vi "Trap2-TestRT-05-16.vi"() -> ()   [LabVIEW 2010]
uses:
  <vilib>/userDefined/High Color/nirio_resource_hc.ctl
  <vilib>/rvi/interface/nirviOpenFPGA/nirviOpenFPGA.xnode
  C:/Users/HAGAR-IV/Desktop/Zeugs/markus/version feb 2012/FPGA Bitfiles/pertrasgcfpga2_FPGATarget_Trap2-Test-05-16_C889B2AB.lvbitx
  C:/Users/HAGAR-IV/Desktop/HAGAR-V_Steuerung/Users/HAGAR-IV/Desktop/Johnny/pertrasgc fpga/Trap2-Test-05-16.vi
  <vilib>/rvi/ClientSDK/nirviWhatTheDeviceIsDoing.ctl
  <vilib>/rvi/interface/nirviReadWriteControl/nirviReadWriteControl.xnode
  <vilib>/rvi/interface/common/niFpgaNodeNameForErrorReporting.ctl
  <vilib>/rvi/errors/niLvFpgaWhatHappensToTopLevelVI.ctl
  <vilib>/rvi/interface/nirviMethod/nirviMethod.xnode
  <vilib>/rvi/interface/nirviCloseFPGA/nirviCloseFPGA.xnode
  <vilib>/FPGAPlugInAG/cRIO-9114/niLvFpga_Open_cRIO-9114.vi
  <vilib>/rvi/interface/common/dynamic/niFpgaDynamicAddResources.vi
  <vilib>/Utility/error.llb/Error Cluster From Error Code.vi
  <vilib>/rvi/errors/niLvFpgaAdjustHostInterfaceError.vi
  <vilib>/FPGAPlugInAG/Dynamic/niLvFpga_Close_Dynamic.vi
  NiFpgaLv.dll
panel:
  out "XY Graph":cluster{dbl[], dbl[]}(graph)
  out "UTempMax":fxp<+/-,16,4> format="%.14g"
  out "UTemp":fxp<+/-,16,4> format="%.14g"
  out "UTempSP":fxp<+/-,16,4> format="%.14g"
  in  "Traps/MachKoeff":dbl[](array[numeric])
  out "UTemp[V]Trap2":dbl format="%.14g"
  in  "stop":bool
  in  "Per[us]Trap2":u32
  in  "warten[us]Trap2":u32
  in  "UTempSPTrap2":dbl format="%.14g"
  in  "UTempMaxTrap2":dbl format="%.14g"
  in  "PIDTrap2":T1 {"proportional gain (Kc)" format="%.11g"; "integral gain (Kc*Ts/Ti)" format="%.11g"; "derivative gain (Kc*Td/Ts)" format="%.11g"}
  in  "Heizen?Trap2":bool
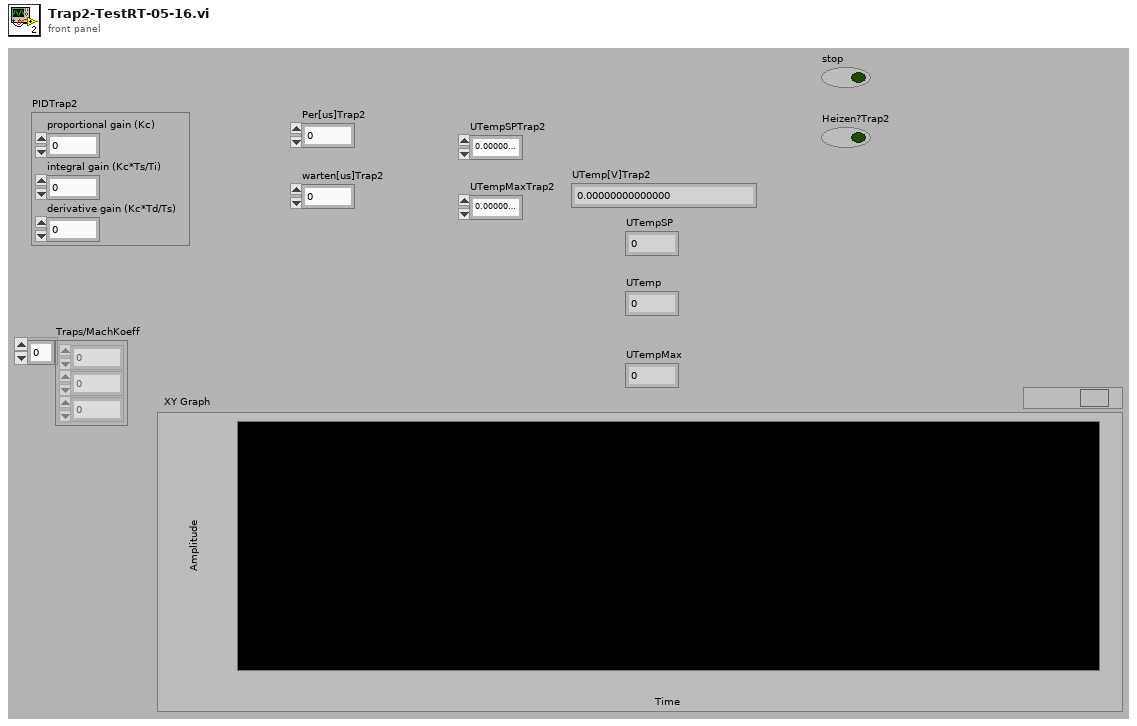
[diagram p1: front panel]
types:
  T1 = cluster{"proportional gain (Kc)":fxp<+/-,16,8>, "integral gain (Kc*Ts/Ti)":fxp<+/-,16,8>, "derivative gain (Kc*Td/Ts)":fxp<+/-,16,8>}
  T2 = typedef "niFpgaNodeNameForErrorReporting.ctl" = enum16{"Open FPGA VI Reference", "Read/Write Control", "Invoke Method: Abort", "Invoke Method: Acknowledge IRQ", "Invoke Method: Download", "Invoke Method: FIFO.Configure", "Invoke Method: FIFO.Read", "Invoke Method: FIFO.Start", "Invoke Method: FIFO.Stop", "Invoke Method: FIFO.Write", "Invoke Method: Reset", "Invoke Method: Run", "Invoke Method: Wait on IRQ", "Close FPGA VI Reference"}
  T3 = typedef "niLvFpgaWhatHappensToTopLevelVI.ctl" = enum16{"top level VI scripted behind XNode", "top level VI inlined behind XNode"}
  T4 = typedef "nirviWhatTheDeviceIsDoing.ctl" = enum32{"nothing", "something other than LabVIEW FPGA", "FPGA interface", "interactive", "emulation"}
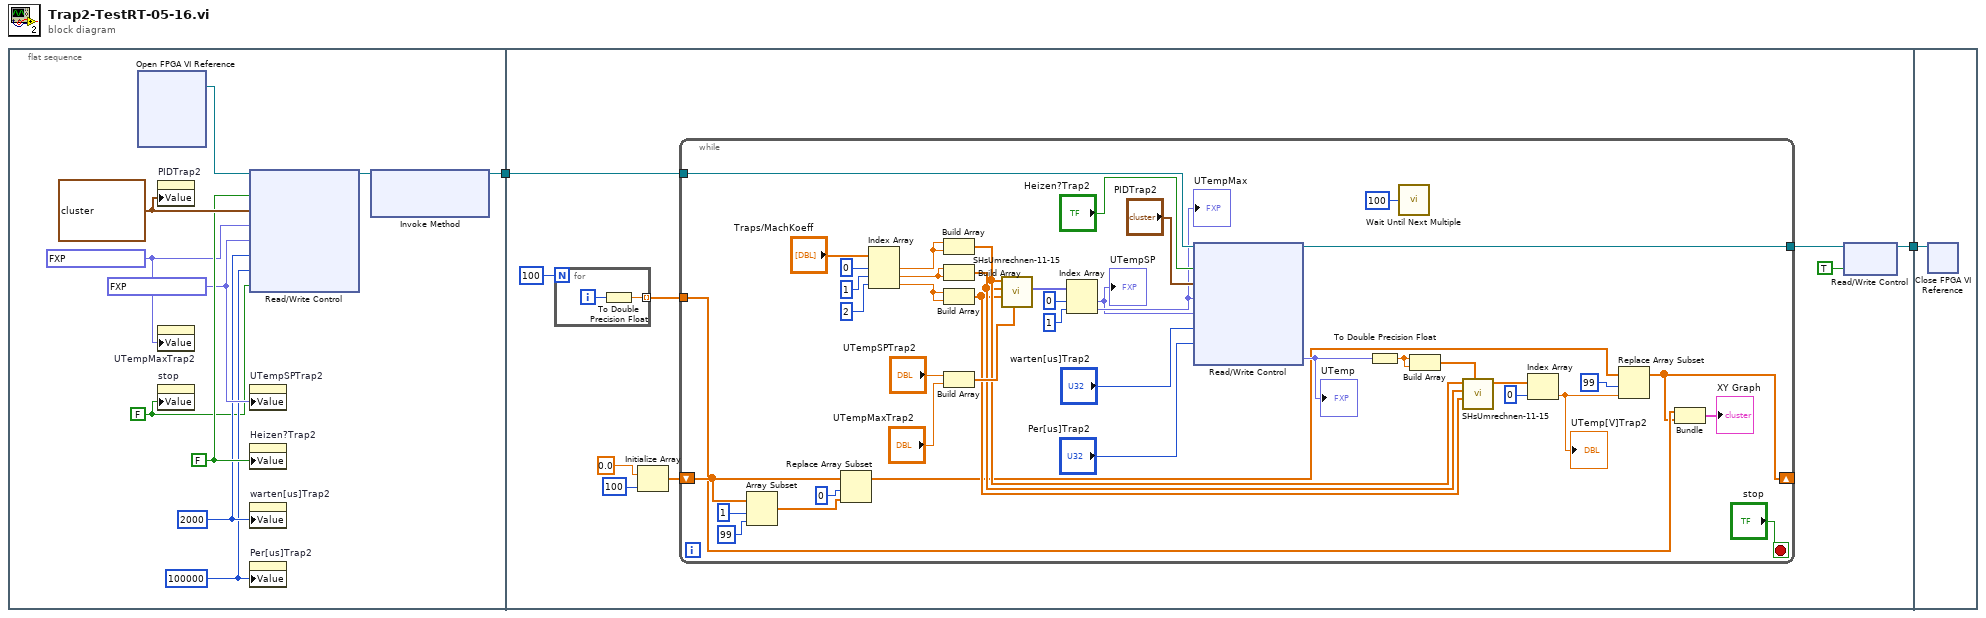
[diagram p0: block diagram]
diagram:
  n1 = flat-sequence {
    tunnel: [w10] -> w2
    tunnel: w2 -> [w304]
    tunnel: [w301] -> w1
    tunnel: w1 -> [w586]
    frame #0 {
      w3 = FALSE ("stop")
      w4 = u32 100000 ("Per[us]Trap2")
      w5 = u32 2000 ("warten[us]Trap2")
      w6 = fxp<+/-,16,4> 0.0 ("UTempSPTrap2")
      w7 = fxp<+/-,16,4> 0.0 ("UTempMaxTrap2")
      w9 = T1 {"proportional gain (Kc)"=0.0, "integral gain (Kc*Ts/Ti)"=0.0, "derivative gain (Kc*Td/Ts)"=0.0} ("PIDTrap2")
      w8 = FALSE ("Heizen?Trap2")
      n2 = xnode "Open FPGA VI Reference"() -> ("FPGA VI Reference Out"=w12:refnum<k20>)  [unwired: 2 in, 1 out]
      n3 = property on="PIDTrap2" class="Clust (strict)"("Value"=w9) -> ()  [unwired: 2 in, 2 out]
      n4 = property on="UTempMaxTrap2" class="DigNum (strict)"("Value"=w7) -> ()  [unwired: 2 in, 2 out]
      n5 = property on="stop" class="Bool (strict)"("Value"=w3) -> ()  [unwired: 2 in, 2 out]
      n6 = xnode "Read/Write Control"("FPGA VI Reference In"=w12, "Heizen?Trap2"=w8, "PIDTrap2"=w9, "UTempMaxTrap2"=w7, "UTempSPTrap2"=w6, "warten[us]Trap2"=w5, "Per[us]Trap2"=w4, "stop"=w3) -> ("FPGA VI Reference Out"=w11:refnum<k20>)  [unwired: 1 in, 1 out]
      n7 = property on="UTempSPTrap2" class="DigNum (strict)"("Value"=w6) -> ()  [unwired: 2 in, 2 out]
      n8 = property on="Heizen?Trap2" class="Bool (strict)"("Value"=w8) -> ()  [unwired: 2 in, 2 out]
      n9 = property on="warten[us]Trap2" class="DigNum (strict)"("Value"=w5) -> ()  [unwired: 2 in, 2 out]
      n10 = property on="Per[us]Trap2" class="DigNum (strict)"("Value"=w4) -> ()  [unwired: 2 in, 2 out]
      n11 = xnode "Invoke Method"("FPGA VI Reference In"=w11) -> ("FPGA VI Reference Out"=w10:refnum<k20>)  [unwired: 2 in, 1 out]
    }
    frame #1 {
      n12 = for {
        N: 100 -> [_]
        tunnel: [w305] -> w296 mode=indexing
        i -> [w306]
        n13 = To Double Precision Float(number=w306) -> (double precision float=w305:dbl)
      }
      n14 = Initialize Array(0.0, 100 ("dimension size")) -> (w298:dbl[])
      n15 = while {
        tunnel: w304 -> [w383]
        tunnel: [w382] -> w303
        shift-right: [w348] -> _
        shift-left: w298 -> [w355]
        tunnel: w296 -> [w349]
        stop <- "stop" stop-if-true
        n16 = Array Subset(array=w355, index=1, length=99) -> (w353:dbl[])
        n17 = Replace Array Subset(array=w355, new element=w353, index=0) -> (w352:dbl[])
        n18 = Index Array(array="Traps/MachKoeff", index #1=0 ("index"), index #2=1 ("index"), index #3=2 ("index")) -> (element #1=w359:dbl, element #2=w360:dbl, element #3=w361:dbl)
        n19 = Build Array(w359, w359) -> (w368:dbl[])
        n20 = Build Array(w360, w360) -> (w367:dbl[])
        n21 = Build Array(w361, w361) -> (w366:dbl[])
        n22 = Build Array("UTempSPTrap2", "UTempMaxTrap2") -> (w378:dbl[])
        n23 = call "SHsUmrechnen-11-15.vi"("TemperaturenSH[V]"=w378, "Traps/MachKoeff2"=w366, "Traps/MachKoeff1"=w367, "Traps/MachKoeff0"=w368) -> ("SpannungenSH[V]"=w377:fxp<+/-,16,4>[])  [unwired: 6 in, 1 out]
        n24 = Index Array(array=w377, index #1=0 ("index"), index #2=1 ("index")) -> (element #1=w363:fxp<+/-,16,4>, element #2=w374:fxp<+/-,16,4>)
        "UTempSP" <- w363
        "UTempMax" <- w374
        n25 = xnode "Read/Write Control"("FPGA VI Reference In"=w383, "Heizen?Trap2"="Heizen?Trap2", "PIDTrap2"="PIDTrap2", "UTempMaxTrap2"=w374, "UTempSPTrap2"=w363, "warten[us]Trap2"="warten[us]Trap2", "Per[us]Trap2"="Per[us]Trap2") -> ("FPGA VI Reference Out"=w382:refnum<k20>, "UTemp[V]Trap2"=w362:fxp<+/-,16,4>)  [unwired: 1 in, 1 out]
        "UTemp" <- w362
        n26 = To Double Precision Float(number=w362) -> (double precision float=w358:dbl)
        n27 = call "Wait Until Next Multiple"("Count(mSec)"=u32 100) -> ()  [unwired: 1 out]
        n28 = Build Array(w358, w358) -> (w369:dbl[])
        n29 = call "SHsUmrechnen-11-15.vi"("SpannungenSH[V]"=w369, "Traps/MachKoeff2"=w366, "Traps/MachKoeff1"=w367, "Traps/MachKoeff0"=w368) -> ("TemperaturenSH[°C]"=w365:dbl[])  [unwired: 6 in, 1 out]
        n30 = Index Array(array=w365, index=0) -> (element=w350:dbl)
        "UTemp[V]Trap2" <- w350
        n31 = Replace Array Subset(array=w352, new element=w350, index=99) -> (w348:dbl[])
        n32 = Bundle(w349, w348) -> (→"XY Graph":cluster{dbl[], dbl[]})  [unwired: 1 in]
      }
      n33 = xnode "Read/Write Control"("FPGA VI Reference In"=w303, "stop"=TRUE) -> ("FPGA VI Reference Out"=w301:refnum<k20>)  [unwired: 1 in, 1 out]
    }
    frame #2 {
      n34 = xnode "Close FPGA VI Reference"("FPGA VI Reference In"=w586) -> ()  [unwired: 1 in, 1 out]
    }
  }
